vi "Start Logic-Mode dependent case 1.vi"(6 "Case name string":string, 8 "error in (no error)":errorcluster, 11 "UI queue":refnum<queue>) -> (0 "error out":errorcluster)   [LabVIEW 2017]
uses:
  Queue/Message Queue/Typedefs/Message Cluster.ctl
  Global Variables/gl_UI Ctrl Refs.vi
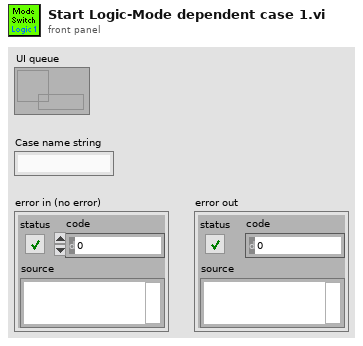
[diagram p1: front panel]
types:
  T1 = typedef "AOL_Globals.ctl" = cluster{"Imaging Protocol":T2, "Number of POI":u16, "Number of Miniscans":u16, "Number of Trials":u16, "Number of Cycles ":u64, "# Averaged Frames":u16, "Laser power (%)":u8, "Pockels (V)":dbl, "Acquisition Length (sec)":dbl, "Fill time (us)":dbl, "POI Dwell time (us)":dbl, "Miniscan Dwell time per pixel (us)":dbl, "PMT 1":dbl, "PMT 2":dbl, "Back Apperture (mA)":dbl, "Frame Size":T3, "Center Frequency":dbl, "Field of View (norm)":dbl, "DwellTime (us)":dbl, "Wavelength (nm)":dbl, "Zoom":dbl, "AOL Z":dbl, "AOL Mode":T4, "GridXY":dbl, "GridZ":dbl, "TriggerPeriod (sec)":dbl, "Number of Pixels in Miniscan":u16, "Experiment folder path":path, "X centre":dbl, "Y centre":dbl, "Angle (degrees)":dbl, "Plane Mode":T5, "Threshold":u16[], "Regenerate Chirps":bool, "Rectangle ROI length (pixels)":u16, "Rectangle ROI height (pixels)":u16, "AOD fill":u16, "StartupDelay":i32, "Samples Wait after Trigger":u16, "Slip Cycle":u32, "Add Cycle":bool, "Functional Mode":T6, "Z Start":dbl, "Z Stop":dbl, "# Planes":i32}
  T2 = typedef "Imaging Protocols enum.ctl" = enum16{"AOL Z-Stack", "Motor Z Stack", "Functional Acquisition", "Single Plane Acquisition", "Volume Acquisition", "Live Imaging", "Live Plane Imaging", "Live Volume Imaging"}
  T3 = typedef "Frame Size.ctl" = u16
  T4 = typedef "AOL modes.ctl" = enum16{"Raster", "Structural", "Pointing", "Mini Scan", "Alignment"}
  T5 = typedef "Plane Mode.ctl" = u16
  T6 = typedef "Functional Mode.ctl" = enum16{"Point", "Line", "Patch", "Plane", "Volume"}
  T7 = typedef "UI ctrl refs cluster.ctl" = cluster{"Top level VI path":path, "Top level VI ref":refnum<vi>, "User menu ref":refnum<k9>, "Sub Panel control":refnum<vi>, "Imaging Param Tab":refnum<vi>, "Occurrence-Start drivers":refnum<k4>, "Occurrence-Speed logging initialised":refnum<k4>, "Occurrence-XYZ stage initialised":refnum<k4>, "Exit button":refnum<vi>, "Status ind":refnum<vi>, "Set as origin":refnum<vi>, "Speed Logging":refnum<vi>, "Time Lapse":refnum<vi>, "Live Imaging":refnum<vi>, "AOL Z Stack":refnum<vi>, "Motor Z Stack":refnum<vi>, "Funct Acq button":refnum<vi>, "Hard Shutter":refnum<vi>, "Virtual Shutter":refnum<vi>, "Laser Power":refnum<vi>, "AOL Mode":refnum<vi>, "Frame Size":refnum<vi>, "Field of View":refnum<vi>, "Dwell Time":refnum<vi>, "Zoom":refnum<vi>, "AOL Z":refnum<vi>, "Objective":refnum<vi>, "Axis":refnum<vi>, "Paths & Names":refnum<vi>, "Experiment folder path (ind.)":refnum<vi>, "Last State (Ind.)":refnum<vi>, "Averages":refnum<vi>, "Angle (degrees)":refnum<vi>, "X centre":refnum<vi>, "Y centre":refnum<vi>, "Plane Mode":refnum<vi>, "# Planes":refnum<vi>, "Z Start":refnum<vi>, "Z Stop":refnum<vi>, "Z Step":refnum<vi>, "PMT 1":refnum<vi>, "PMT 2":refnum<vi>, "Stage XYZ Position":refnum<vi>, "Pockels@Z Start":refnum<vi>, "Pockels@Z Stop":refnum<vi>, "Obtain Z Start":refnum<vi>, "Obtain Z Stop":refnum<vi>, "Live stim.trig.period":refnum<vi>, "Live stim.trig.enable":refnum<vi>, "Movement Correction":refnum<vi>, "Load Reference Image":refnum<vi>, "XY Stage Move":refnum<vi>, "MovCor Cluster":refnum<vi>, "RefDAQParam":refnum<vi>, "Funct. Acq. Pockels Modulation":refnum<vi>, "Ref Laser Power":refnum<vi>, "Enable Video Recording":refnum<vi>, "Video Record-Live Imaging":refnum<vi>, "Video Record-Funct acq":refnum<vi>, "Reference Source":refnum<vi>, "AOL Z-stack Chirps Ready (ind)":refnum<vi>, "Target time between mov.cor. ref triggers (ms)":refnum<vi>, "Funct. Acq. Ref frame save":refnum<vi>, "Tracking button":refnum<vi>, "Show ref plots window":refnum<vi>, "Center freq ind (nm)":refnum<vi>, "Pickup mode (ind)":refnum<vi>, "Logging queue (ind)":refnum<vi>, "Back aperture power (ind.)":refnum<vi>, "Power after objective (ind.)":refnum<vi>, "Switch user":refnum<vi>, "Ls1 Conn. Status":refnum<vi>, "Ls1Tuning Status":refnum<vi>, "Ls1 Faults":refnum<vi>, "Ls1 Connection":refnum<vi>, "Ls1 Mode":refnum<vi>, "Ls1 POWER [mW]":refnum<vi>, "Ls1Shutter":refnum<vi>, "Ls1 Wavelength":refnum<vi>, "Ls1 Note":refnum<vi>, "Ls1 Confirm Wav":refnum<vi>, "Ls1 PreChrp Prism1":refnum<vi>, "Ls1 PreChrp Prism2":refnum<vi>, "Ls1 wav top Ind":refnum<vi>, "Ls1 power top Ind":refnum<vi>, "Ls1 Pump peak Hold":refnum<vi>, "Ls1 Status Ind":refnum<vi>, "Ls1 wav cancel":refnum<vi>, "Experiment Type":refnum<vi>, "Biology Information":refnum<vi>}
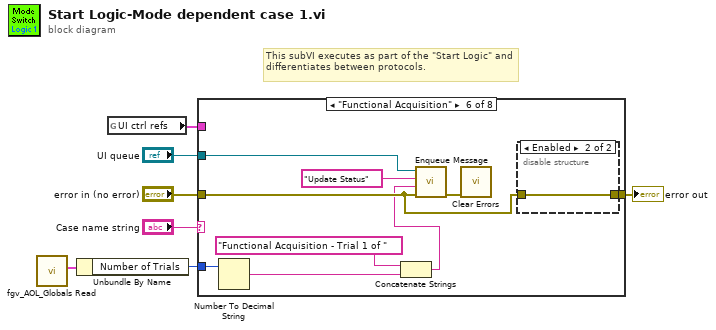
[diagram p0: block diagram]
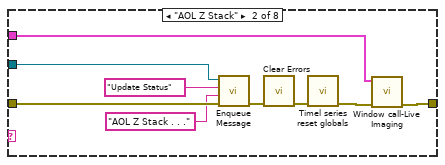
[diagram p3: hidden frame]
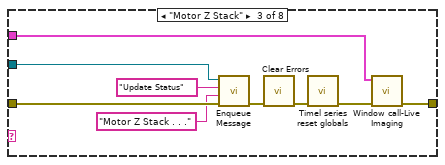
[diagram p4: hidden frame]
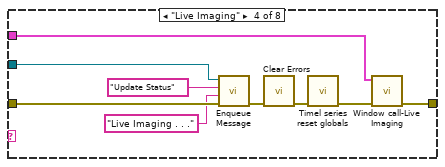
[diagram p5: hidden frame]
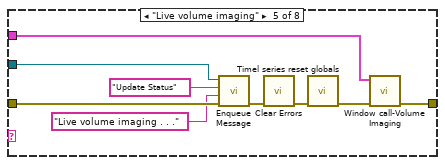
[diagram p6: hidden frame]
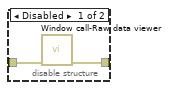
[diagram p7: hidden frame]
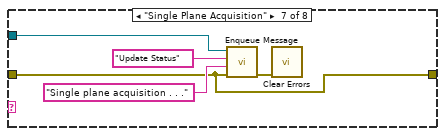
[diagram p8: hidden frame]
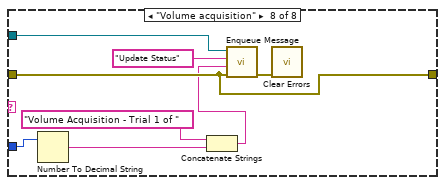
[diagram p9: hidden frame]
diagram:
  # "This subVI executes as part of the \"Start Logic\" and differentiates between protocols."
  n1 = call "fgv_AOL_Globals Read.vi"() -> ("AOL_Globals"=w2:T1)  [unwired: 9 in, 2 out]
  n2 = Unbundle By Name(w2) -> ("Number of Trials"=w1:u16)
  n3 = global read "gl_UI Ctrl Refs.vi" "UI ctrl refs"() -> (w4:T7)
  n4 = case shown="\"Functional Acquisition\"" "Case name string" {
    tunnel: "error in (no error)" -> [w8 w17 w26 w35 w44 w50 w57 w66]
    tunnel: "UI queue" -> [_ w16 w25 w34 w43 w53 w61 w69]
    tunnel: w4 -> [_ w10 w19 w28 w37 _ _ _]
    tunnel: [w8 w9 w18 w27 w36 w49 w57 w66] -> w3
    tunnel: w1 -> [_ _ _ _ _ w48 _ w62]
    frame Default {
    }
    frame "AOL Z Stack" {
      n5 = call "Enqueue Message.vi"("error in (no error)"=w17, "Message Data"="AOL Z Stack . . ." ("Acquiring and Logging..."), "Message"="Update Status", "Queue"=w16) -> ("error out"=w14:errorcluster)  [unwired: 6 in, 1 out]
      n6 = call <vilib>:"Clear Errors.vi"("error in (no error)"=w14) -> ("error out"=w12:errorcluster)  [unwired: 5 in, 1 out]
      n7 = call "Timel series reset globals.vi"("error in (no error)"=w12) -> ("error out"=w11:errorcluster)  [unwired: 10 in]
      n8 = call "Window call-Live Imaging.vi"("error in (no error)"=w11, "UI ctrl refs"=w10) -> ("error out"=w9:errorcluster)  [unwired: 9 in]
    }
    frame "Motor Z Stack" {
      n9 = call "Enqueue Message.vi"("error in (no error)"=w26, "Message Data"="Motor Z Stack . . ." ("Acquiring and Logging..."), "Message"="Update Status", "Queue"=w25) -> ("error out"=w23:errorcluster)  [unwired: 6 in, 1 out]
      n10 = call <vilib>:"Clear Errors.vi"("error in (no error)"=w23) -> ("error out"=w21:errorcluster)  [unwired: 5 in, 1 out]
      n11 = call "Timel series reset globals.vi"("error in (no error)"=w21) -> ("error out"=w20:errorcluster)  [unwired: 10 in]
      n12 = call "Window call-Live Imaging.vi"("error in (no error)"=w20, "UI ctrl refs"=w19) -> ("error out"=w18:errorcluster)  [unwired: 9 in]
    }
    frame "Live Imaging" {
      n13 = call "Enqueue Message.vi"("error in (no error)"=w35, "Message Data"="Live Imaging . . ." ("Acquiring and Logging..."), "Message"="Update Status", "Queue"=w34) -> ("error out"=w32:errorcluster)  [unwired: 6 in, 1 out]
      n14 = call <vilib>:"Clear Errors.vi"("error in (no error)"=w32) -> ("error out"=w30:errorcluster)  [unwired: 5 in, 1 out]
      n15 = call "Timel series reset globals.vi"("error in (no error)"=w30) -> ("error out"=w29:errorcluster)  [unwired: 10 in]
      n16 = call "Window call-Live Imaging.vi"("error in (no error)"=w29, "UI ctrl refs"=w28) -> ("error out"=w27:errorcluster)  [unwired: 9 in]
    }
    frame "Live volume imaging" {
      n17 = call "Enqueue Message.vi"("error in (no error)"=w44, "Message Data"="Live volume imaging . . ." ("Acquiring and Logging..."), "Message"="Update Status", "Queue"=w43) -> ("error out"=w41:errorcluster)  [unwired: 6 in, 1 out]
      n18 = call <vilib>:"Clear Errors.vi"("error in (no error)"=w41) -> ("error out"=w39:errorcluster)  [unwired: 5 in, 1 out]
      n19 = call "Timel series reset globals.vi"("error in (no error)"=w39) -> ("error out"=w38:errorcluster)  [unwired: 10 in]
      n20 = call "Window call-Volume Imaging.vi"("error in (no error)"=w38, "UI ctrl refs"=w37) -> ("error out"=w36:errorcluster)  [unwired: 9 in]
    }
    frame "Functional Acquisition" {
      n21 = Number To Decimal String(number=w48) -> (decimal integer string=w46:string)  [unwired: 1 in]
      n22 = Concatenate Strings("Functional Acquisition - Trial 1 of " ("Acquiring and Logging..."), w46) -> (w45:string)
      n23 = call "Enqueue Message.vi"("error in (no error)"=w50, "Message Data"=w45, "Message"="Update Status", "Queue"=w53) -> ("error out"=w51:errorcluster)  [unwired: 6 in, 1 out]
      n24 = call <vilib>:"Clear Errors.vi"("error in (no error)"=w51) -> ()  [unwired: 5 in, 2 out]
      n25 = disable-structure shown="Enabled" {
        disable-tunnel: w50 -> [w55 w56]
        disable-tunnel: [w54 w56] -> w49
        frame Disabled {
          n26 = call "Window call-Raw data viewer.vi"("error in (no error)"=w55) -> ("error out"=w54:errorcluster)  [unwired: 10 in]
        }
        frame Enabled {
        }
      }
    }
    frame "Single Plane Acquisition" {
      n27 = call "Enqueue Message.vi"("error in (no error)"=w57, "Message Data"="Single plane acquisition . . ." ("Acquiring and Logging..."), "Message"="Update Status", "Queue"=w61) -> ("error out"=w59:errorcluster)  [unwired: 6 in, 1 out]
      n28 = call <vilib>:"Clear Errors.vi"("error in (no error)"=w59) -> ()  [unwired: 5 in, 2 out]
    }
    frame "Volume acquisition" {
      n29 = Number To Decimal String(number=w62) -> (decimal integer string=w64:string)  [unwired: 1 in]
      n30 = Concatenate Strings("Volume Acquisition - Trial 1 of " ("Acquiring and Logging..."), w64) -> (w63:string)
      n31 = call "Enqueue Message.vi"("error in (no error)"=w66, "Message Data"=w63, "Message"="Update Status", "Queue"=w69) -> ("error out"=w67:errorcluster)  [unwired: 6 in, 1 out]
      n32 = call <vilib>:"Clear Errors.vi"("error in (no error)"=w67) -> ()  [unwired: 5 in, 2 out]
    }
  }
  "error out" <- w3
